vi "GetActualDriveDistance.vi"(8 "Robot Motion Commands In":T1, 9 "Zero Encoder":bool) -> (3 "Robot Motion Commands Out":T1)   [LabVIEW 2019]
uses:
  Controls/Robot Pivot Motion Commands.ctl
  Controls/Pivot Motor Commands.ctl
  Controls/Robot Drive Mode.ctl
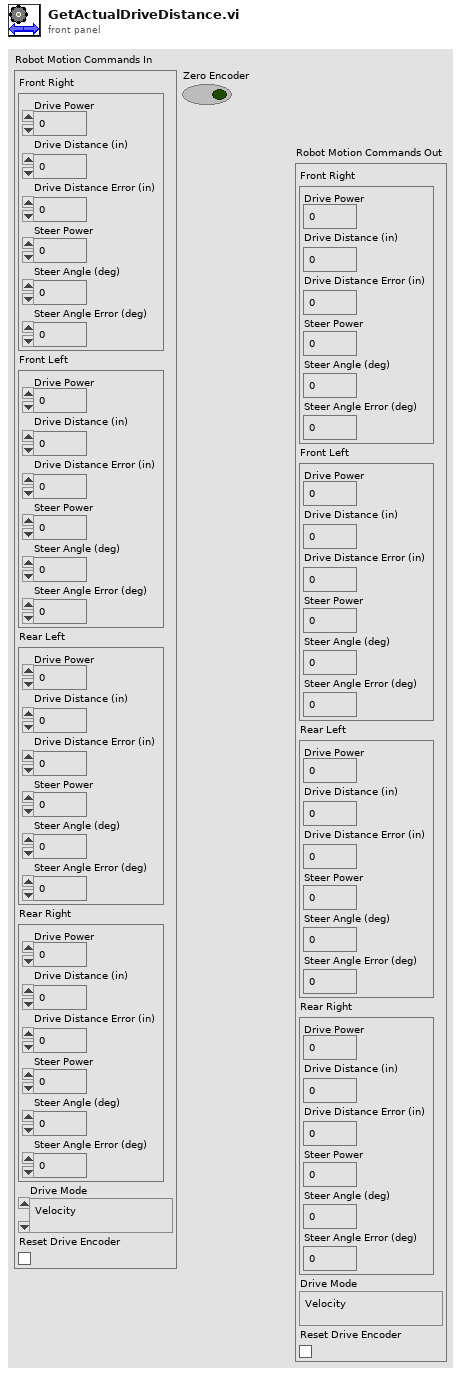
[diagram p1: front panel]
types:
  T1 = typedef "Robot Pivot Motion Commands.ctl" = cluster{"Front Right":T2, "Front Left":T2, "Rear Left":T2, "Rear Right":T2, "Drive Mode":T3, "Reset Drive Encoder":bool}
  T2 = typedef "Pivot Motor Commands.ctl" = cluster{"Drive Power":dbl, "Drive Distance (in)":dbl, "Drive Distance Error (in)":dbl, "Steer Power":dbl, "Steer Angle (deg)":dbl, "Steer Angle Error (deg)":dbl}
  T3 = typedef "Robot Drive Mode.ctl" = enum16{"Velocity", "Distance"}
  T4 = typedef "WPI_EncoderDevRef.ctl" = cluster{"DevStatus":errorcluster, "EncoderIndex":T5, "CounterIndex":T6, "DistancePerCount":dbl, "Decoding Type":T7}
  T5 = typedef "FPGA_EncoderIdx.ctl" = enum8{"Enc 0", "Enc 1", "Enc 2", "Enc 3", "Enc 4", "Enc 5", "Enc 6", "Enc 7", "Invalid"}
  T6 = typedef "FPGA_CounterCtrSystemIndex.ctl" = enum8{"Ctr 0", "Ctr 1", "Ctr 2", "Ctr 3", "Ctr 4", "Ctr 5", "Ctr 6", "Ctr 7", "Invalid"}
  T7 = typedef "WPI_EncoderType.ctl" = enum16{"1x", "2x", "4x"}
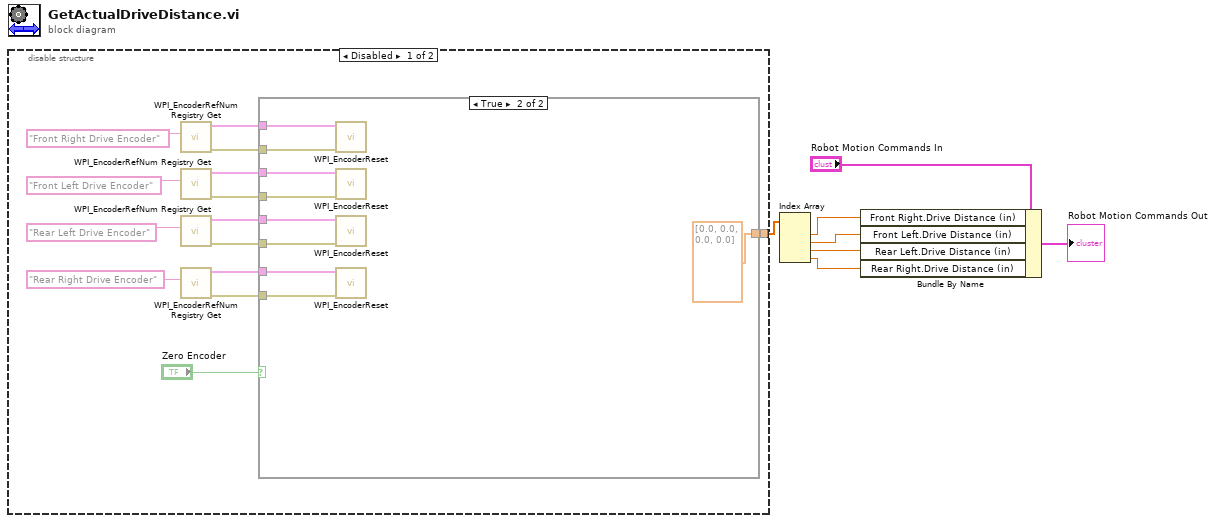
[diagram p0: block diagram]
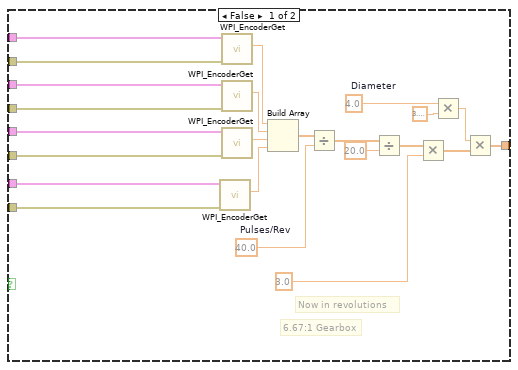
[diagram p2: hidden frame]
diagram:
  n1 = disable-structure shown="Disabled" {
    disable-tunnel: [w21 _] -> w5
    frame Disabled {
      n2 = call <vilib>:"WPI_EncoderRefNum Registry Get.vi"("refnum name"="Front Right Drive Encoder") -> ("error out"=w10:errorcluster, "EncoderDevRef"=w9:T4)  [unwired: 9 in]
      n3 = call <vilib>:"WPI_EncoderRefNum Registry Get.vi"("refnum name"="Front Left Drive Encoder") -> ("error out"=w12:errorcluster, "EncoderDevRef"=w11:T4)  [unwired: 9 in]
      n4 = call <vilib>:"WPI_EncoderRefNum Registry Get.vi"("refnum name"="Rear Left Drive Encoder") -> ("error out"=w14:errorcluster, "EncoderDevRef"=w13:T4)  [unwired: 9 in]
      n5 = call <vilib>:"WPI_EncoderRefNum Registry Get.vi"("refnum name"="Rear Right Drive Encoder") -> ("error out"=w16:errorcluster, "EncoderDevRef"=w15:T4)  [unwired: 9 in]
      n6 = case shown="True" "Zero Encoder" {
        tunnel: [w30 dbl[] [0.0, 0.0, 0.0, 0.0]] -> w21
        tunnel: w16 -> [w29 w45]
        tunnel: w15 -> [w28 w46]
        tunnel: w14 -> [w27 w47]
        tunnel: w13 -> [w26 w48]
        tunnel: w12 -> [w25 w49]
        tunnel: w11 -> [w24 w50]
        tunnel: w10 -> [w23 w51]
        tunnel: w9 -> [w22 w52]
        frame False {
          w41 = 4.0  # Diameter
          w44 = 40.0  # Pulses/Rev
          # "Now in revolutions"
          # "6.67:1 Gearbox"
          n7 = call <vilib>:"WPI_EncoderGet.vi"("error in (no error)"=w29, "EncoderDevRef"=w28) -> ("Distance"=w32:dbl)  [unwired: 4 in, 5 out]
          n8 = call <vilib>:"WPI_EncoderGet.vi"("error in (no error)"=w23, "EncoderDevRef"=w22) -> ("Distance"=w35:dbl)  [unwired: 4 in, 5 out]
          n9 = call <vilib>:"WPI_EncoderGet.vi"("error in (no error)"=w25, "EncoderDevRef"=w24) -> ("Distance"=w34:dbl)  [unwired: 4 in, 5 out]
          n10 = call <vilib>:"WPI_EncoderGet.vi"("error in (no error)"=w27, "EncoderDevRef"=w26) -> ("Distance"=w33:dbl)  [unwired: 4 in, 5 out]
          n11 = Build Array(w35, w34, w33, w32) -> (w31:dbl[])
          n12 = Divide(x=w31, y=w44) -> (x/y=w43:dbl[])
          n13 = Divide(x=w43, y=20.0) -> (x/y=w38:dbl[])
          n14 = Multiply(x=w38, y=3.0) -> (x*y=w37:dbl[])
          n15 = Multiply(x=w41, y=3.141592653589793) -> (x*y=w39:dbl)
          n16 = Multiply(x=w39, y=w37) -> (x*y=w30:dbl[])
        }
        frame True {
          n17 = call <vilib>:"WPI_EncoderReset.vi"("error in (no error)"=w51, "EncoderDevRef"=w52) -> ()  [unwired: 8 in, 2 out]
          n18 = call <vilib>:"WPI_EncoderReset.vi"("error in (no error)"=w49, "EncoderDevRef"=w50) -> ()  [unwired: 8 in, 2 out]
          n19 = call <vilib>:"WPI_EncoderReset.vi"("error in (no error)"=w47, "EncoderDevRef"=w48) -> ()  [unwired: 8 in, 2 out]
          n20 = call <vilib>:"WPI_EncoderReset.vi"("error in (no error)"=w45, "EncoderDevRef"=w46) -> ()  [unwired: 8 in, 2 out]
        }
      }
    }
    frame Enabled {
    }
  }
  n21 = Index Array(array=w5) -> (element #1=w4:dbl, element #2=w3:dbl, element #3=w2:dbl, element #4=w1:dbl)  [unwired: 4 in]
  n22 = Bundle By Name(cluster="Robot Motion Commands In", "Front Right.Drive Distance (in)"=w4, "Front Left.Drive Distance (in)"=w3, "Rear Left.Drive Distance (in)"=w2, "Rear Right.Drive Distance (in)"=w1) -> (→"Robot Motion Commands Out":T1)
